vi "backwards difference (dbl).vi"(3 "Y":dbl[](array[numeric])) -> (1 "Y(i)-Y(i-1)":dbl[](array[numeric]))   [LabVIEW 2009, in "common.lvlib"]
uses:
  common.lvlib
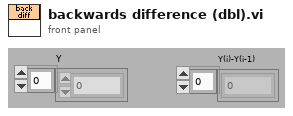
[diagram p1: front panel]
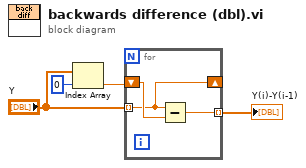
[diagram p0: block diagram]
diagram:
  n1 = Index Array(array="Y", index=0) -> (element=w2:dbl)
  n2 = for {
    tunnel: "Y" -> [w6] mode=indexing
    shift-right: [w6] -> _
    shift-left: w2 -> [w7]
    tunnel: [w5] -> w1 mode=indexing
    n3 = Subtract(x=w6, y=w7) -> (x-y=w5:dbl)
  }
  "Y(i)-Y(i-1)" <- w1
